vi "Scannig-Probe-Microscope-Controller-2010-03-08-RFR-1a-version-for-MCL-drift-trial-fm-multiple-channels-nanoh50.vi"() -> ()   [LabVIEW 2012]
uses:
  <vilib>/rvi/eio/common/nirviEmuTemplateMethod_errors.vi
  <vilib>/rvi/Emulation/niFpgaSctlEmulationGetInTimedLoop.vi
  <vilib>/rvi/Emulation/niFpgaSctlEmulationGlobalWrite.vi
  <vilib>/rvi/interface/RandomDataEmulation/nirviRandomDataFPGAFIFO.vi
  <vilib>/rvi/interface/RandomDataEmulation/niFpgaRandomDataHandleErrors.vi
  <vilib>/eio/EIONode/EIONode.xnode
  <vilib>/rvi/Analysis/measure/butterworth/XNode/niFpgaButterworthFilter.xnode
  <vilib>/rvi/DataTransferAndStorage/Container/XNode/niFpgaContainer.xnode
  <vilib>/rvi/interface/RandomDataEmulation/nirviRandomDataFpgaReadWriteTemplate.vi
panel:
  in  "P scale":i8=-1
  in  "Setpoint Control":bool
  in  "Internal Setpoint Internal Control":i16
  in  "Internal Setpoint External Control":i16=357
  in  "Stop Feedback Control":bool
  in  "shift integrator":i32
  out "offset out":i16
  in  "drift temporal control":u32
  out "TF-drift":i16
  out "Counter Data":i8 min=-1 step=1
  out "End of image":bool
  in  "Pixels in one image":i32
  in  "Scanning Y indicator":bool
  in  "Steps per Feedback Region":i32=665
  in  "Y Number of Lines":u32=10
  in  "PID gains (x 2^8)":T1={"proportional gain (Kc)"=1, "integral gain (Kc*Ts/Ti)"=0, "derivative gain (Kc*Td/Ts)"=0}
  out "Command Out":i16=-4104
  in  "provisional limit":i8=102
  out "accumulator limit":i8=-1
  in  "shift-divisions (always >=2)":i8=100
  out "limit indicator":u8
  in  "counter":i8 min=-1 step=1
  in  "Internal Setpoint":i16=357
  in  "I scale":i8=-1
  in  "Count(uSec)":u8=232
  in  "Timeout FIFO":i32=-1
  out "Y line":i32
  out "iterations x":i32
  out "X Output Value":i16=3
  in  "Forth/Back Y axis":bool
  out "Inidicator \nforth/back  Y axis":i8=1
  in  "Time per step/\nX axis sub pixel (uSec)":u16=31 caption="Count(uSec)"
  in  "Time per image pixel/\nX axis pixel (uSec)":u16=1984 caption="Count(uSec)"
  in  "Time per step/\nY axis sub pixel (uSec)":u32=7936 caption="Count(uSec)"
  out "Y Output Value":i16=32702
  out "End of scan line?":bool
  in  "Forth/Back X axis":bool
  in  "Image Total Pixels":u32=65536
  out "Indicator \nforth/back X axis":i8=1
  in  "Y axis pixels":u16=255
  in  "Y steps per pixel":u16=64
  in  "X steps per pixel":u16=64
  in  "y initial":i16
  in  "x initial":i16
  in  "X axis pixels":u16=255
  in  "Scanning On/Off":bool
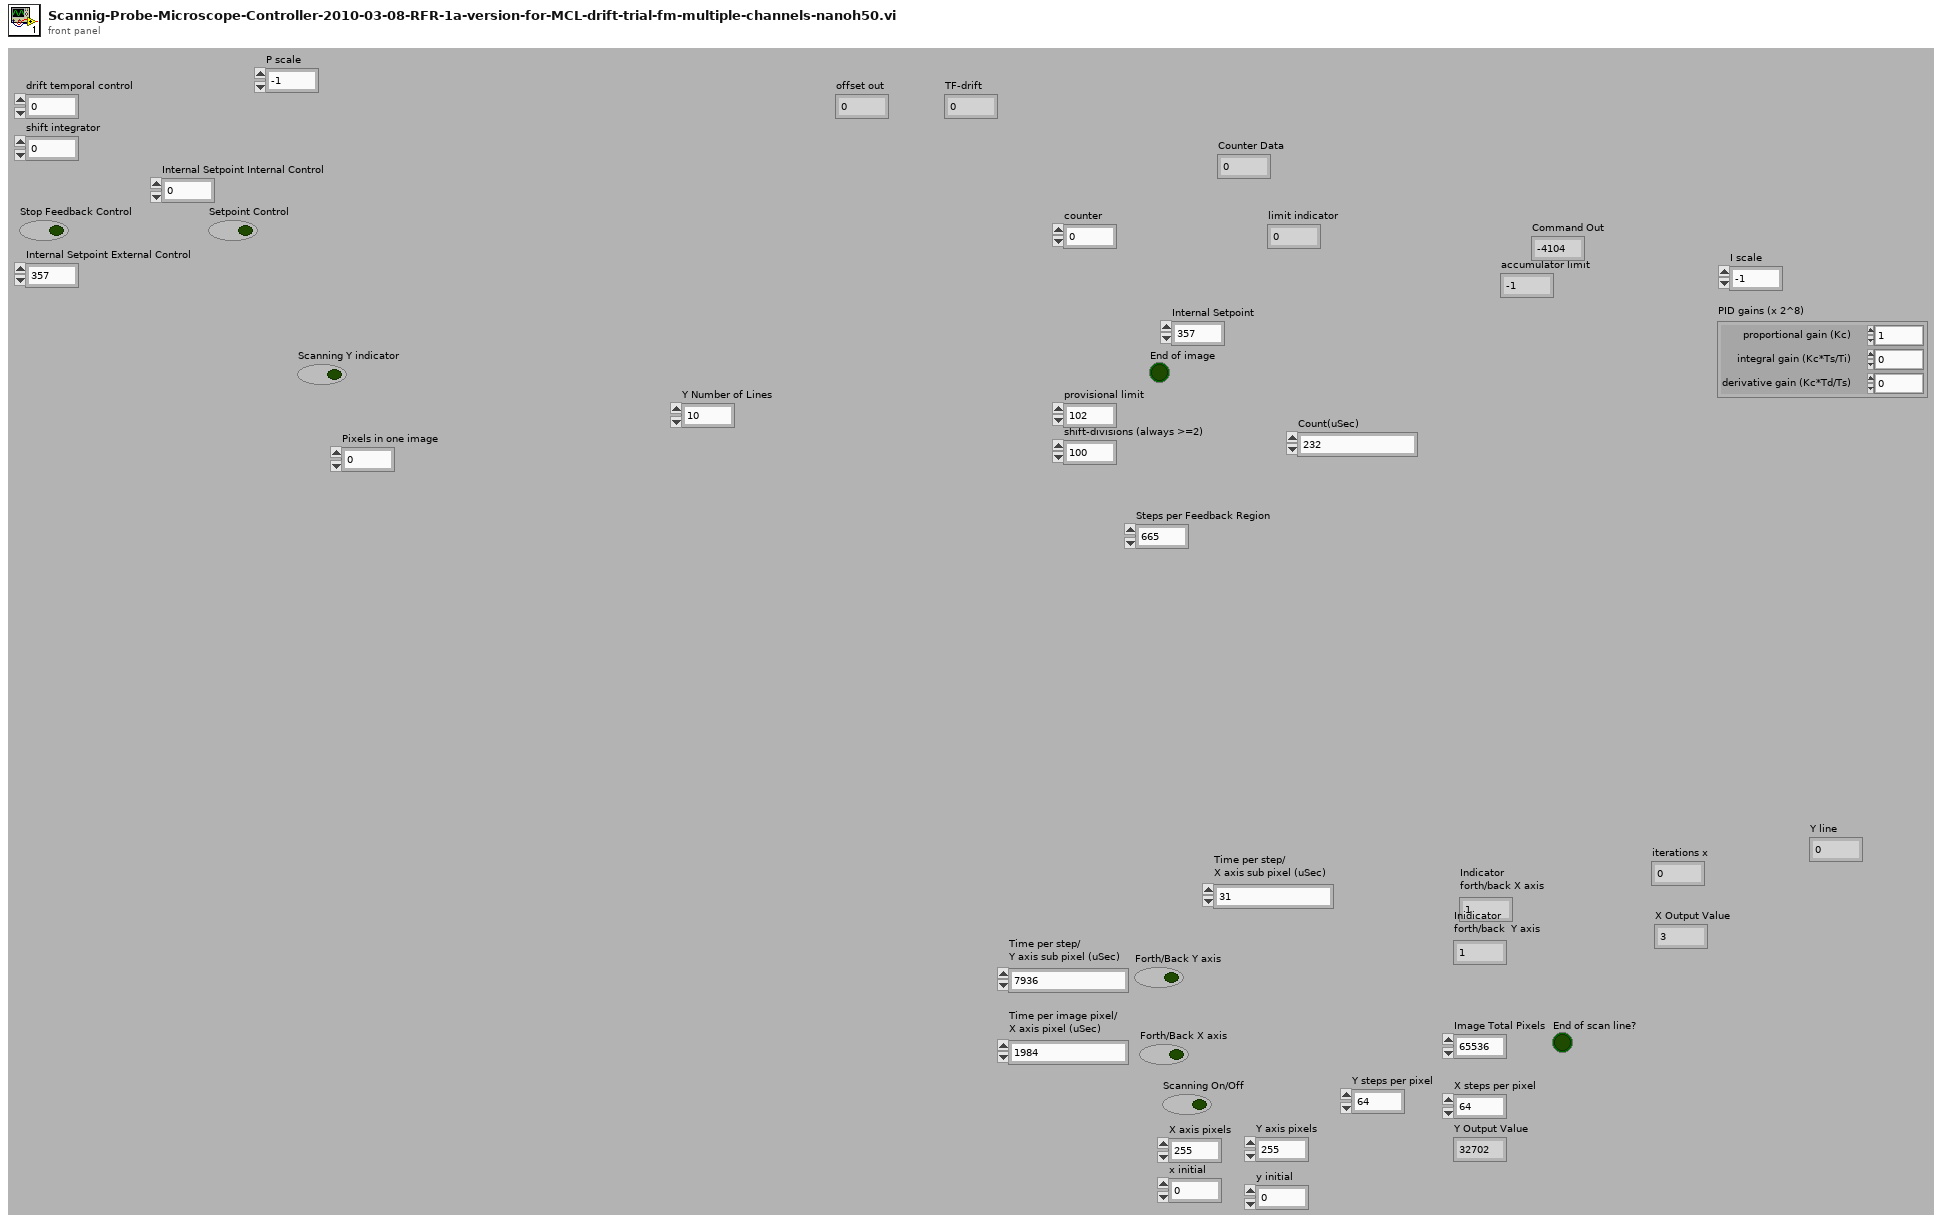
[diagram p1: front panel]
types:
  T1 = cluster{"proportional gain (Kc)":i16, "integral gain (Kc*Ts/Ti)":i16, "derivative gain (Kc*Td/Ts)":i16}
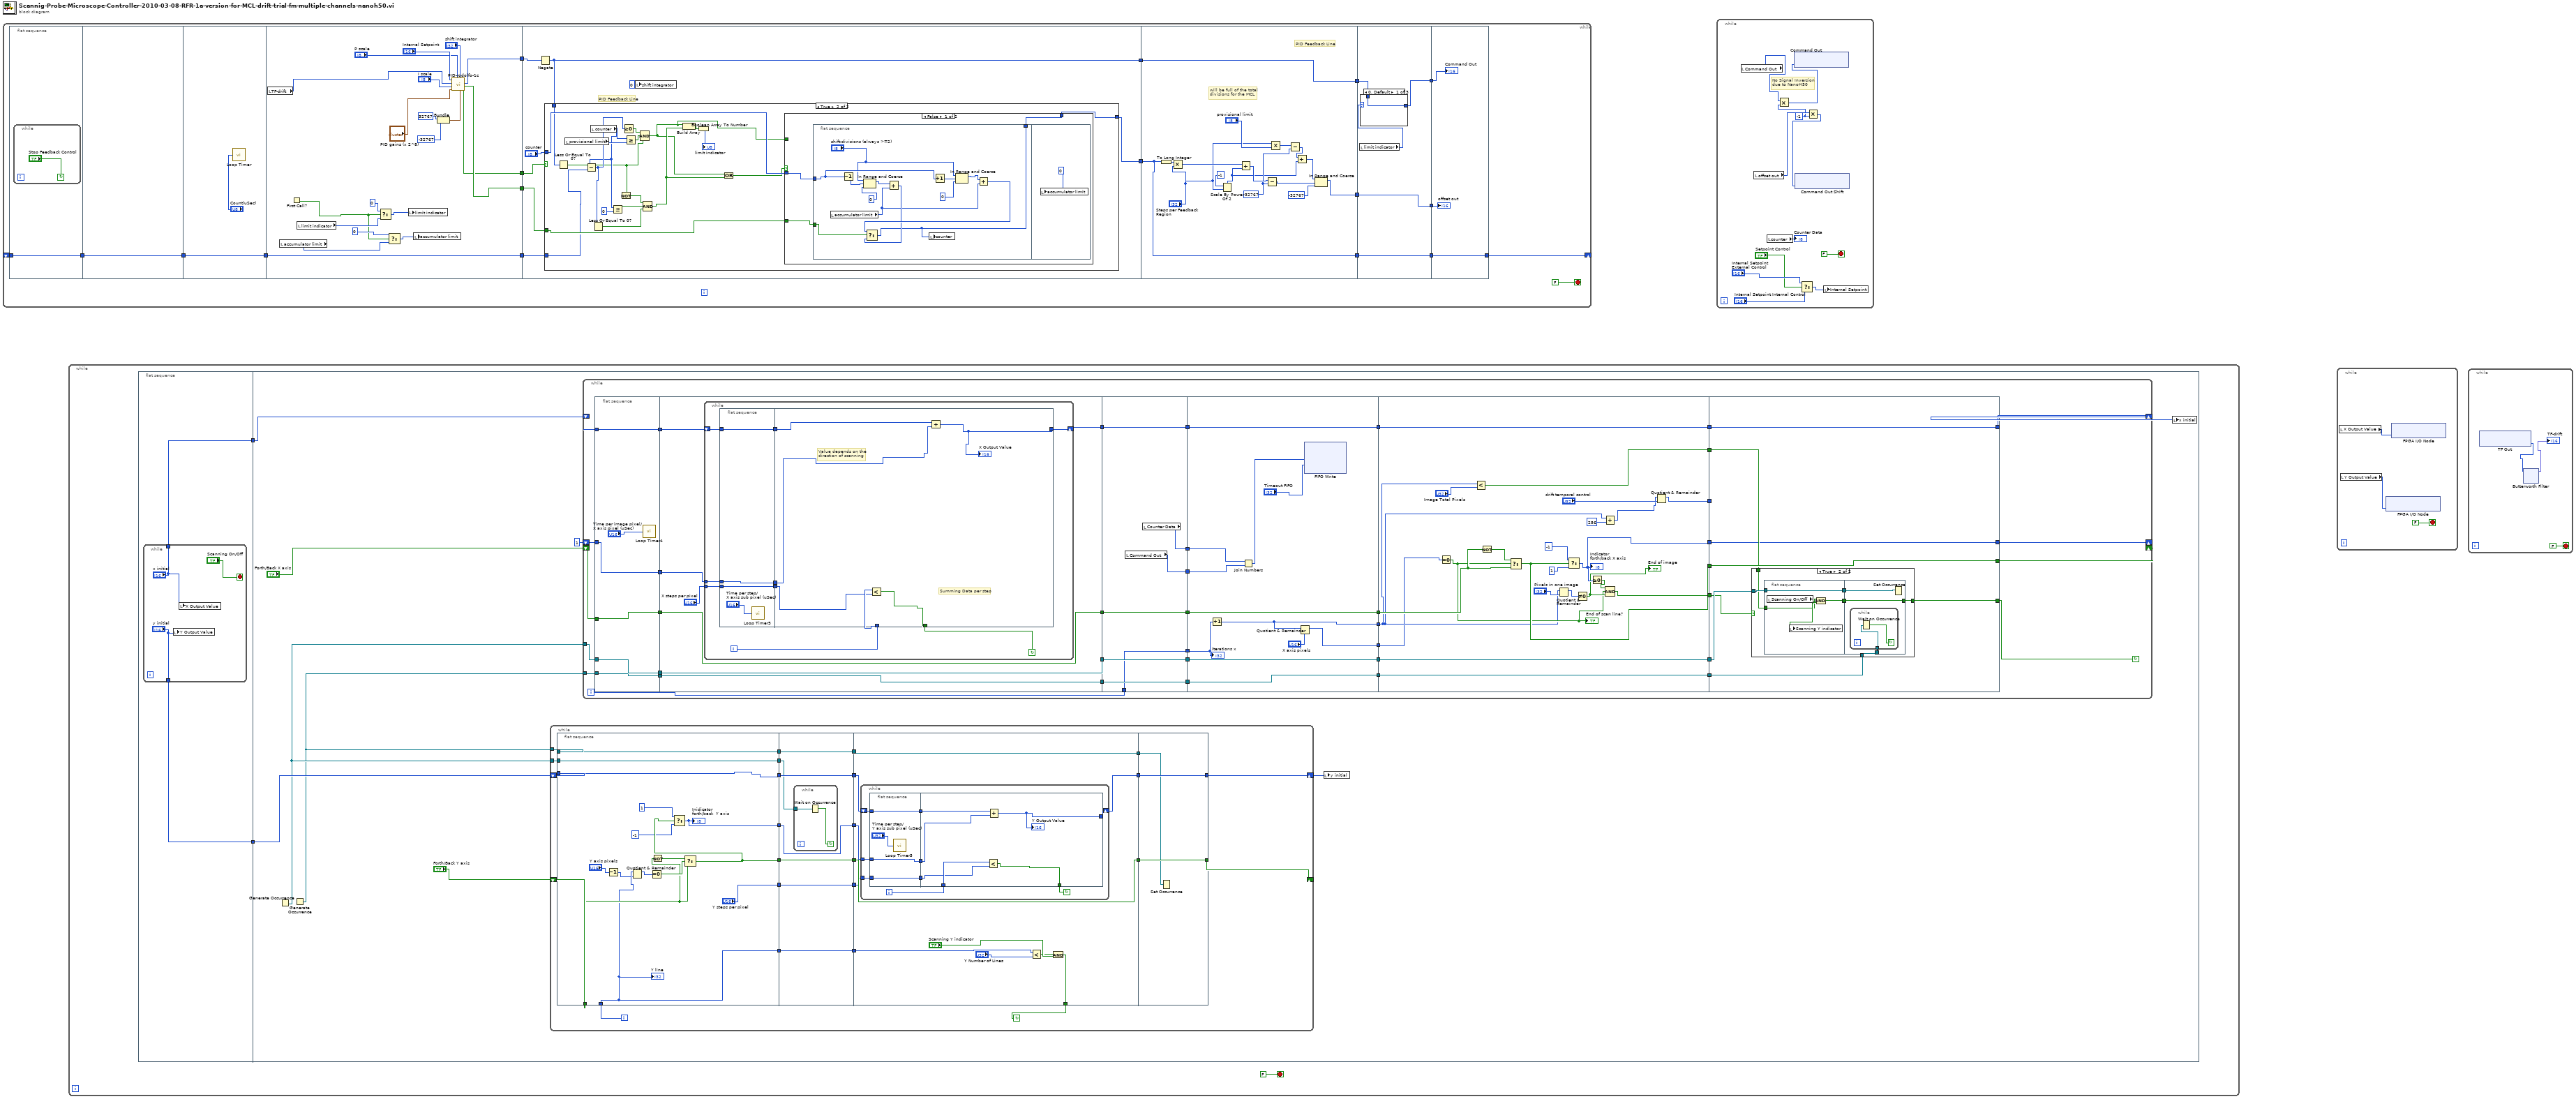
[diagram p0: block diagram]
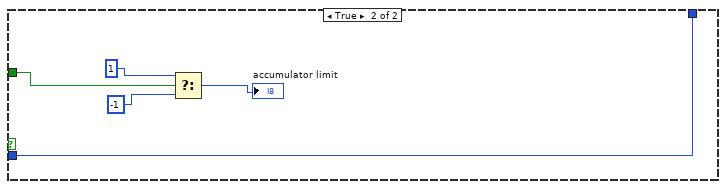
[diagram p3: hidden frame]
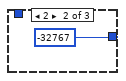
[diagram p4: hidden frame]
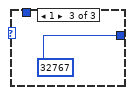
[diagram p5: hidden frame]
diagram:
  n1 = while {
    shift-right: [w9] -> _
    shift-left: _ -> [w8]
    stop <- FALSE stop-if-true
    n2 = flat-sequence {
      tunnel: w8 -> [w19]
      tunnel: [w19] -> w2
      tunnel: w2 -> [w21]
      tunnel: [w21] -> w1
      tunnel: [w22] -> w7
      tunnel: w1 -> [w22]
      tunnel: [w40] -> w6
      tunnel: [w39] -> w5
      tunnel: [w38] -> w4
      tunnel: w7 -> [w35]
      tunnel: [w35] -> w3
      tunnel: [w51] -> w12
      tunnel: w6 -> [w50]
      tunnel: [w46] -> w13
      tunnel: w5 -> [w48]
      tunnel: w4 -> [w47]
      tunnel: w3 -> [w45]
      tunnel: w13 -> [w108]
      tunnel: [w108] -> w15
      tunnel: w12 -> [w105]
      tunnel: [w106] -> w14
      tunnel: [w105] -> w11
      tunnel: [w112] -> w17
      tunnel: w15 -> [w114]
      tunnel: [w115] -> w16
      tunnel: w14 -> [w112]
      tunnel: w11 -> [w111]
      tunnel: [w111] -> w10
      tunnel: w17 -> [w119]
      tunnel: w16 -> [w121]
      tunnel: w10 -> [w120]
      tunnel: [w120] -> w9
      frame #0 {
        n3 = while {
          stop <- "Stop Feedback Control" continue-if-true
        }
      }
      frame #1 {
      }
      frame #2 {
        n4 = call "Loop Timer"("Count(uSec)"="Count(uSec)") -> ()  [unwired: 1 out]
      }
      frame #3 {
        n5 = local read "TF-drift"() -> (w25:i16)
        n6 = local read "accumulator limit"() -> (w28:i8)
        n7 = First Call?() -> (First Call?: T/F=w26:bool)
        n8 = local read "limit indicator"() -> (w31:u8)
        n9 = Select(t=u8 0, s=w26, f=w31) -> (s? t:f=w32:u8)
        n10 = Select(t=i8 0, s=w26, f=w28) -> (s? t:f=w30:i8)
        n11 = local write "limit indicator"(w32) -> ()
        n12 = local write "accumulator limit"(w30) -> ()
        n13 = Bundle(i16 32767, i16 -32767) -> (w41:cluster{i16, i16})  [unwired: 1 in]
        n14 = call "PID-rodolfo-1c.vi"("output range"=w41, "shift integrator"="shift integrator", "P scale"="P scale", "PID gains (x 2^8)"="PID gains (x 2^8)", "I scale"="I scale", "process variable"=w25, "setpoint"="Internal Setpoint") -> ("yes/no"=w38:bool, "upper/lower"=w39:bool, "output"=w40:i16)  [unwired: 2 in]
      }
      frame #4 {
        # "PID Feedback Line"
        n15 = Negate(x=w50) -> (-x=w46:i16)
        n16 = case shown="True" w47 {
          tunnel: "counter" -> [w52 w72]
          tunnel: [w52 w71] -> w51
          tunnel: w48 -> [_ w55]
          tunnel: w46 -> [_ w60]
          tunnel: w45 -> [_ w53]
          frame False {
          }
          frame True {
            n17 = Less Or Equal To 0?(x=w60) -> (x <= 0?=w61:bool)
            n18 = local read "provisional limit"() -> (w68:i8)
            n19 = local read "counter"() -> (w63:i8)
            n20 = Subtract(x=w63, y=w53) -> (x-y=w64:i8)
            n21 = Less Or Equal To 0?(x=w64) -> (x <= 0?=w65:bool)
            n22 = Less Or Equal?(x=w63, y=u8 0) -> (x <= y?=w66:bool)
            n23 = Not(x=w61) -> (.not. x?=w62:bool)
            n24 = Greater Or Equal To 0?(x=w64) -> (x >= 0?=w70:bool)
            n25 = Greater Or Equal?(x=w63, y=w68) -> (x >= y?=w69:bool)
            n26 = Compound Arithmetic op=AND(w70, w69, w61) -> (w54:bool)
            n27 = Compound Arithmetic op=AND(w62, w66, w65) -> (w57:bool)
            n28 = Build Array(w54, w57) -> (w59:bool[])
            n29 = Boolean Array To Number(Boolean array=w59) -> (number=→"limit indicator":u8)
            n30 = Or(x=w54, y=w57) -> (x .or. y?=w56:bool)
            n31 = case shown="False" w56 {
              tunnel: w72 -> [w75 w94]
              tunnel: [w74 w94] -> w71
              tunnel: w55 -> [w73 _]
              tunnel: w54 -> [_ w90]
              frame False {
                n32 = flat-sequence {
                  tunnel: w75 -> [w81]
                  tunnel: [w78] -> w74
                  tunnel: w73 -> [w82]
                  frame #0 {
                    n33 = local read "accumulator limit"() -> (w77:i8)
                    n34 = Decrement(x=w81) -> (x-1=w85:i8)
                    n35 = In Range and Coerce(upper limit="shift-divisions (always >=2)", x=w85, lower limit=i8 0) -> (coerced(x)=w83:i8)  [unwired: 1 out]
                    n36 = Add(x=w83, y=w77) -> (x+y=w79:i8)
                    n37 = Increment(x=w81) -> (x+1=w86:i8)
                    n38 = In Range and Coerce(upper limit="shift-divisions (always >=2)", x=w86, lower limit=i8 0 ("y")) -> (coerced(x)=w88:i8)  [unwired: 1 out]
                    n39 = Add(x=w88, y=w77) -> (x+y=w80:i8)
                    n40 = Select(t=w80, s=w82, f=w79) -> (s? t:f=w78:i8)
                    n41 = local write "counter"(w78) -> ()
                  }
                  frame #1 {
                    n42 = local write "accumulator limit"(i8 0 ("accumulator limit")) -> ()
                  }
                }
              }
              frame True {
                n43 = Select(t=i8 1, s=w90, f=i8 -1) -> (s? t:f=→"accumulator limit":i8)
              }
            }
          }
        }
        n44 = local write "shift integrator"(0 ("new integrator")) -> ()
      }
      frame #5 {
        w98 = 32767 ("y")
        # "PID Feedback Line"
        # "will be full of the total\ndivisions for the MCL"
        n45 = To Long Integer(number=w105) -> (32bit integer=w104:i32)
        n46 = Multiply(x=w104, y="Steps per Feedback Region") -> (x*y=w109:i32)
        n47 = Scale By Power Of 2(n=i8 -1, x="Steps per Feedback Region") -> (x*2^n=w97:i32)
        n48 = Add(x=w109, y=w97) -> (x+y=w101:i32)
        n49 = Subtract(x=w101, y=w98) -> (x-y=w100:i32)
        n50 = Multiply(x="Steps per Feedback Region", y="provisional limit") -> (x*y=w99:i32)
        n51 = Subtract(x=w99, y=w98) -> (x-y=w96:i32)
        n52 = Add(x=w96, y=w97) -> (x+y=w95:i32)
        n53 = In Range and Coerce(upper limit=w95, x=w100, lower limit=-32767) -> (coerced(x)=w106:i32)  [unwired: 1 out]
      }
      frame #6 {
        n54 = local read "limit indicator"() -> (w113:u8)
        n55 = case shown="0, Default" w113 {
          tunnel: w114 -> [w116 _ _]
          tunnel: [w116 i16 -32767 i16 32767] -> w115
          frame 0, Default {
          }
          frame 2 {
          }
          frame 1 {
          }
        }
      }
      frame #7 {
        "Command Out" <- w121
        "offset out" <- w119
      }
    }
  }
  n56 = while {
    stop <- FALSE stop-if-true
    n57 = flat-sequence {
      tunnel: [w125] -> w123
      tunnel: [w126] -> w122
      tunnel: w123 -> [w134]
      tunnel: w122 -> [w133]
      frame #0 {
        n58 = while {
          tunnel: ["y initial"] -> w126
          tunnel: ["x initial"] -> w125
          stop <- "Scanning On/Off" stop-if-true
          n59 = local write "Y Output Value"("y initial") -> ()
          n60 = local write "X Output Value"("x initial") -> ()
        }
      }
      frame #1 {
        n61 = Generate Occurrence() -> (w132:refnum<k4>)
        n62 = Generate Occurrence() -> (w131:refnum<k4>)
        n63 = while {
          shift-right: [w162] -> _
          shift-left: "Forth/Back Y axis" -> [w161]
          shift-right: [w159] -> w135
          shift-left: w133 -> [w160]
          tunnel: w132 -> [w158]
          tunnel: w131 -> [w154]
          i -> [w142]
          stop <- w141 continue-if-true
          n64 = flat-sequence {
            tunnel: w161 -> [w175]
            tunnel: [w173] -> w153
            tunnel: [w170] -> w151
            tunnel: [w169] -> w149
            tunnel: [w168] -> w147
            tunnel: ["Y steps per pixel"] -> w145
            tunnel: [w166] -> w143
            tunnel: w142 -> [w165]
            tunnel: w160 -> [w170]
            tunnel: w154 -> [w168]
            tunnel: w158 -> [w166]
            tunnel: [w165] -> w139
            tunnel: w153 -> [w184]
            tunnel: [w184] -> w152
            tunnel: w151 -> [w183]
            tunnel: [w183] -> w150
            tunnel: w149 -> [w182]
            tunnel: [w182] -> w148
            tunnel: w147 -> [w181]
            tunnel: [w181] -> w146
            tunnel: w145 -> [w180]
            tunnel: [w180] -> w144
            tunnel: w143 -> [w179]
            tunnel: [w178] -> w140
            tunnel: w139 -> [w178]
            tunnel: w152 -> [w197]
            tunnel: w150 -> [w196]
            tunnel: w148 -> [w194]
            tunnel: [w197] -> w157
            tunnel: [w195] -> w156
            tunnel: [w193] -> w155
            tunnel: w146 -> [w193]
            tunnel: w144 -> [w192]
            tunnel: [w188] -> w141
            tunnel: w140 -> [w187]
            tunnel: [w218] -> w159
            tunnel: [w219] -> w162
            tunnel: w157 -> [w219]
            tunnel: w156 -> [w218]
            tunnel: w155 -> [w217]
            frame #0 {
              n65 = Decrement(x="Y axis pixels") -> (x-1=w163:u16)
              n66 = Quotient & Remainder(x=w165, y=w163) -> (x-y*floor(x/y)=w177:i32)  [unwired: 1 out]
              n67 = Equal To 0?(x=w177) -> (x = 0?=w176:bool)
              n68 = Not(x=w175) -> (.not. x?=w174:bool)
              n69 = Select(t=w174, s=w176, f=w175) -> (s? t:f=w173:bool)
              n70 = Select(t=i8 1, s=w173, f=i8 -1 ("Inidicator \nforth/back  Y axis")) -> (s? t:f=w169:i8)
              "Inidicator \nforth/back  Y axis" <- w169
              "Y line" <- w165
            }
            frame #1 {
              n71 = while {
                tunnel: w179 -> [w185]
                stop <- w186 continue-if-true
                n72 = Wait on Occurrence(2:w185) -> (0:w186:bool)  [unwired: 2 in]
              }
            }
            frame #2 {
              n73 = while {
                shift-right: [w203] -> w195
                shift-left: w196 -> [w204]
                tunnel: w194 -> [w200]
                tunnel: w192 -> [w198]
                i -> [w205]
                stop <- w206 continue-if-true
                n74 = flat-sequence {
                  tunnel: w204 -> [w210]
                  tunnel: [w210] -> w202
                  tunnel: [w208] -> w201
                  tunnel: w200 -> [w208]
                  tunnel: [w207] -> w199
                  tunnel: w198 -> [w207]
                  tunnel: [w212] -> w206
                  tunnel: w205 -> [w216]
                  tunnel: [w214] -> w203
                  tunnel: w202 -> [w215]
                  tunnel: w201 -> [w213]
                  tunnel: w199 -> [w211]
                  frame #0 {
                    n75 = call "Loop Timer5"("Count(uSec)"="Time per step/\nY axis sub pixel (uSec)") -> ()  [unwired: 1 out]
                  }
                  frame #1 {
                    n76 = Less?(x=w216, y=w211) -> (x < y?=w212:bool)
                    n77 = Add(x=w215, y=w213) -> (x+y=w214:i16)
                    "Y Output Value" <- w214
                  }
                }
              }
              n78 = Less?(x=w187, y="Y Number of Lines") -> (x < y?=w189:bool)
              n79 = Compound Arithmetic op=AND(w189, "Scanning Y indicator") -> (w188:bool)
            }
            frame #3 {
              n80 = Set Occurrence(w217) -> ()
            }
          }
        }
        n81 = while {
          shift-right: [w257] -> w136
          shift-left: w134 -> [w259]
          shift-right: [w244] -> _
          shift-left: "Forth/Back X axis" -> [w258]
          tunnel: w132 -> [w256]
          tunnel: w131 -> [w255]
          shift-right: [w246] -> _
          shift-left: i8 1 ("Indicator \nforth/back") -> [w245]
          i -> [w226]
          stop <- w254 continue-if-true
          n82 = flat-sequence {
            tunnel: w258 -> [w264]
            tunnel: w259 -> [w265]
            tunnel: [w265] -> w243
            tunnel: [w264] -> w242
            tunnel: w256 -> [w262]
            tunnel: [w262] -> w241
            tunnel: [w261] -> w240
            tunnel: w255 -> [w261]
            tunnel: [w260] -> w239
            tunnel: w245 -> [w260]
            tunnel: w243 -> [w270]
            tunnel: [w272] -> w238
            tunnel: [w269] -> w234
            tunnel: w240 -> [w269]
            tunnel: [w268] -> w232
            tunnel: w241 -> [w268]
            tunnel: [w267] -> w230
            tunnel: w242 -> [w267]
            tunnel: w239 -> [w271]
            tunnel: w238 -> [w298]
            tunnel: [w298] -> w237
            tunnel: [w293] -> w236
            tunnel: [w294] -> w235
            tunnel: w234 -> [w297]
            tunnel: [w297] -> w233
            tunnel: w232 -> [w296]
            tunnel: [w296] -> w231
            tunnel: w230 -> [w295]
            tunnel: [w295] -> w229
            tunnel: [w292] -> w227
            tunnel: w226 -> [w292]
            tunnel: w237 -> [w310]
            tunnel: w236 -> [w309]
            tunnel: w235 -> [w305]
            tunnel: [w310] -> w225
            tunnel: [w308] -> w224
            tunnel: w233 -> [w308]
            tunnel: [w307] -> w223
            tunnel: w231 -> [w307]
            tunnel: [w306] -> w222
            tunnel: w229 -> [w306]
            tunnel: w227 -> [w304]
            tunnel: [w302] -> w221
            tunnel: [w301] -> w220
            tunnel: [w325] -> w253
            tunnel: w225 -> [w333]
            tunnel: [w333] -> w252
            tunnel: w224 -> [w332]
            tunnel: [w332] -> w251
            tunnel: w223 -> [w331]
            tunnel: [w331] -> w250
            tunnel: [w326] -> w249
            tunnel: w222 -> [w324]
            tunnel: [w323] -> w248
            tunnel: [w322] -> w247
            tunnel: [w315] -> w228
            tunnel: w221 -> [w312]
            tunnel: w220 -> [w311]
            tunnel: [w340] -> w257
            tunnel: [w341] -> w244
            tunnel: w253 -> [w341]
            tunnel: w252 -> [w340]
            tunnel: w251 -> [w339]
            tunnel: w250 -> [w338]
            tunnel: w249 -> [w337]
            tunnel: [w336] -> w254
            tunnel: w248 -> [w335]
            tunnel: [w334] -> w246
            tunnel: w247 -> [w334]
            tunnel: w228 -> [_]
            frame #0 {
              n83 = call "Loop Timer4"("Count(uSec)"="Time per image pixel/\nX axis pixel (uSec)") -> ()  [unwired: 1 out]
            }
            frame #1 {
              n84 = while {
                shift-right: [w278] -> w272
                shift-left: w270 -> [w279]
                tunnel: w271 -> [w275]
                tunnel: "X steps per pixel" -> [w273]
                i -> [w280]
                stop <- w281 continue-if-true
                n85 = flat-sequence {
                  tunnel: w279 -> [w285]
                  tunnel: [w285] -> w277
                  tunnel: [w283] -> w276
                  tunnel: w275 -> [w283]
                  tunnel: [w282] -> w274
                  tunnel: w273 -> [w282]
                  tunnel: [w287] -> w281
                  tunnel: w280 -> [w291]
                  tunnel: [w289] -> w278
                  tunnel: w277 -> [w290]
                  tunnel: w276 -> [w288]
                  tunnel: w274 -> [w286]
                  frame #0 {
                    n86 = call "Loop Timer3"("Count(uSec)"="Time per step/\nX axis sub pixel (uSec)") -> ()  [unwired: 1 out]
                  }
                  frame #1 {
                    # "Summing Data per step"
                    # "Value depends on the\ndirection of scanning"
                    n87 = Less?(x=w291, y=w286) -> (x < y?=w287:bool)
                    n88 = Add(x=w290, y=w288) -> (x+y=w289:i16)
                    "X Output Value" <- w289
                  }
                }
              }
            }
            frame #2 {
              n89 = local read "Command Out"() -> (w294:i16)
              n90 = local read "Counter Data"() -> (w293:i8)
            }
            frame #3 {
              n91 = Increment(x=w304) -> (x+1=w302:i32)
              n92 = Join Numbers(hi=w309, lo=w305) -> ((hi.lo)=w299:u32)
              n93 = Quotient & Remainder(x=w302, y="X axis pixels") -> (x-y*floor(x/y)=w301:i32)  [unwired: 1 out]
              n94 = xnode "FIFO Write"("Element"=w299, "Timeout"="Timeout FIFO") -> ()  [unwired: 1 in, 2 out]
              "iterations x" <- w304
            }
            frame #4 {
              n95 = Equal To 0?(x=w311) -> (x = 0?=w318:bool)
              "End of scan line?" <- w318
              n96 = Less?(x=w312, y="Image Total Pixels") -> (x < y?=w326:bool)
              n97 = Not(x=w324) -> (.not. x?=w330:bool)
              n98 = Select(t=w330, s=w318, f=w324) -> (s? t:f=w325:bool)
              n99 = Quotient & Remainder(x=w312, y="Pixels in one image") -> (x-y*floor(x/y)=w319:i32)  [unwired: 1 out]
              n100 = Select(t=i8 -1 ("Indicator \nforth/back"), s=w325, f=i8 1 ("Indicator \nforth/back")) -> (s? t:f=w322:i8)
              "Indicator \nforth/back X axis" <- w322
              n101 = Not Equal To 0?(x=w319) -> (x != 0?=w321:bool)
              "End of image" <- w321
              n102 = Greater Or Equal To 0?(x=w322) -> (x >= 0?=w317:bool)
              n103 = Add(x=w312, y=u16 256) -> (x+y=w313:i32)
              n104 = Compound Arithmetic op=AND(w317, w318, w321) -> (w323:bool)
              n105 = Quotient & Remainder(x=w313, y="drift temporal control") -> (x-y*floor(x/y)=w315:u32)  [unwired: 1 out]
            }
            frame #5 {
              n106 = case shown="True" w335 {
                tunnel: w338 -> [_ w348]
                tunnel: w339 -> [_ w347]
                tunnel: w337 -> [w342 w345]
                tunnel: [w342 w344] -> w336
                frame False {
                }
                frame True {
                  n107 = flat-sequence {
                    tunnel: w348 -> [w352]
                    tunnel: [w352] -> w346
                    tunnel: w345 -> [w350]
                    tunnel: [w349] -> w343
                    tunnel: w347 -> [w354]
                    tunnel: w346 -> [w355]
                    tunnel: [w353] -> w344
                    tunnel: w343 -> [w353]
                    frame #0 {
                      n108 = local read "Scanning On/Off"() -> (w351:bool)
                      n109 = local write "Scanning Y indicator"(w351) -> ()
                      n110 = Compound Arithmetic op=AND(w350, w351) -> (w349:bool)
                    }
                    frame #1 {
                      n111 = while {
                        tunnel: w354 -> [w356]
                        stop <- w357 continue-if-true
                        n112 = Wait on Occurrence(2:w356) -> (0:w357:bool)  [unwired: 2 in]
                      }
                      n113 = Set Occurrence(w355) -> ()
                    }
                  }
                }
              }
            }
          }
        }
        n114 = local write "y initial"(w135) -> ()
        n115 = local write "x initial"(w136) -> ()
      }
    }
  }
  n116 = while {
    stop <- FALSE stop-if-true
    w359 = i16 -1 ("y")
    # "No Signal Inversion\ndue to NanoH50"
    n117 = local read "Command Out"() -> (w362:i16)
    n118 = local read "offset out"() -> (w361:i16)
    n119 = local read "counter"() -> (→"Counter Data":i8)
    n120 = Multiply(x=w362, y=w359) -> (x*y=w358:i16)
    n121 = xnode "Command Out"("Connector0/AO7"=w358) -> ()  [unwired: 1 in, 1 out]
    n122 = Select(t="Internal Setpoint External Control", s="Setpoint Control", f="Internal Setpoint Internal Control") -> (s? t:f=w365:i16)
    n123 = Multiply(x=w361, y=w359) -> (x*y=w360:i16)
    n124 = xnode "Command Out Shift"("Connector0/AO2"=w360) -> ()  [unwired: 1 in, 1 out]
    n125 = local write "Internal Setpoint"(w365) -> ()
  }
  n126 = while {
    stop <- FALSE stop-if-true
    n127 = local read "X Output Value"() -> (w370:i16)
    n128 = local read "Y Output Value"() -> (w369:i16)
    n129 = xnode "FPGA I/O Node"("Connector0/AO3"=w369) -> ()  [unwired: 1 in, 1 out]
    n130 = xnode "FPGA I/O Node"("Connector0/AO0"=w370) -> ()  [unwired: 1 in, 1 out]
  }
  n131 = while {
    stop <- FALSE stop-if-true
    n132 = xnode "TF Out"() -> ("Connector0/AI7"=w373:i16)  [unwired: 1 in, 1 out]
    n133 = xnode "Butterworth Filter"("input data"=w373) -> ("output data"=→"TF-drift":fxp<+/-,20,20>)  [unwired: 2 in]
  }
